vi "Protection Channel.vi"(8 "error in (no error)":errorcluster, 11 "Node Ptr":T2 format="%.0x") -> (0 "error out":errorcluster)   [LabVIEW 2015, in "J1939 Addon System Explorer.lvlib"]
uses:
  J1939 Addon System Explorer.lvlib
  <vilib>/NI Veristand/Custom Device API/Custom Device Item Ref.ctl
  Protection Support/Source/Shared/Types/Protection Type.ctl
  <vilib>/NI VeriStand/Custom Device API/Custom Device API.lvlib
  Protection Support/Source/System Explorer/Protection and Counter Support System Explorer.lvlib
  Protection Support/Source/Shared/Protection and Counter Support Shared.lvlib
panel:
  in  "Protection Type":T1
  in  "SHDocVw.IWebBrowser":refnum<k7>(container)
  in  "Monitored Channels":i32(listbox)
  in  "Header":cluster{"Section Name":string}={"Section Name"="Custom Device Item Settings"}
  in  "Description":string
  in  "Name":string
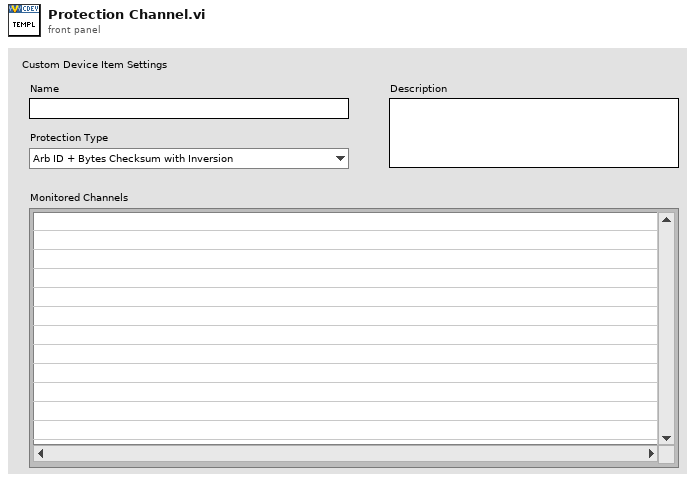
[diagram p1: front panel]
types:
  T1 = typedef "Protection and Counter Support Shared.lvlib/Protection Type.ctl" = enum16{"Arb ID + Bytes Checksum with Inversion", "Arb ID + Bytes CRC with Inversion", "Reversed Raw Signal Checksum with Inversion"}
  T2 = typedef "Custom Device API.lvlib/Custom Device Item Ref.ctl" = u64
  T3 = typedef "Custom Device API.lvlib/Custom Device Item Info.ctl" = cluster{"Name":string, "Is Channel":bool, "GUID":string, "Is Waveform":bool}
  T4 = typedef "Protection and Counter Support System Explorer.lvlib/Protection Signal Settings.ctl" = cluster{"Input Channels":T5[], "Protection Type":T1}
  T5 = typedef "Protection and Counter Support System Explorer.lvlib/Protection Signal Linked Channel.ctl" = cluster{"Node Ref":T2}
  T6 = typedef "Custom Device API.lvlib/Custom Device Commands.ctl" = enum16{"Default", "Item renamed", "Shutdown", "Dynamic button pressed"}
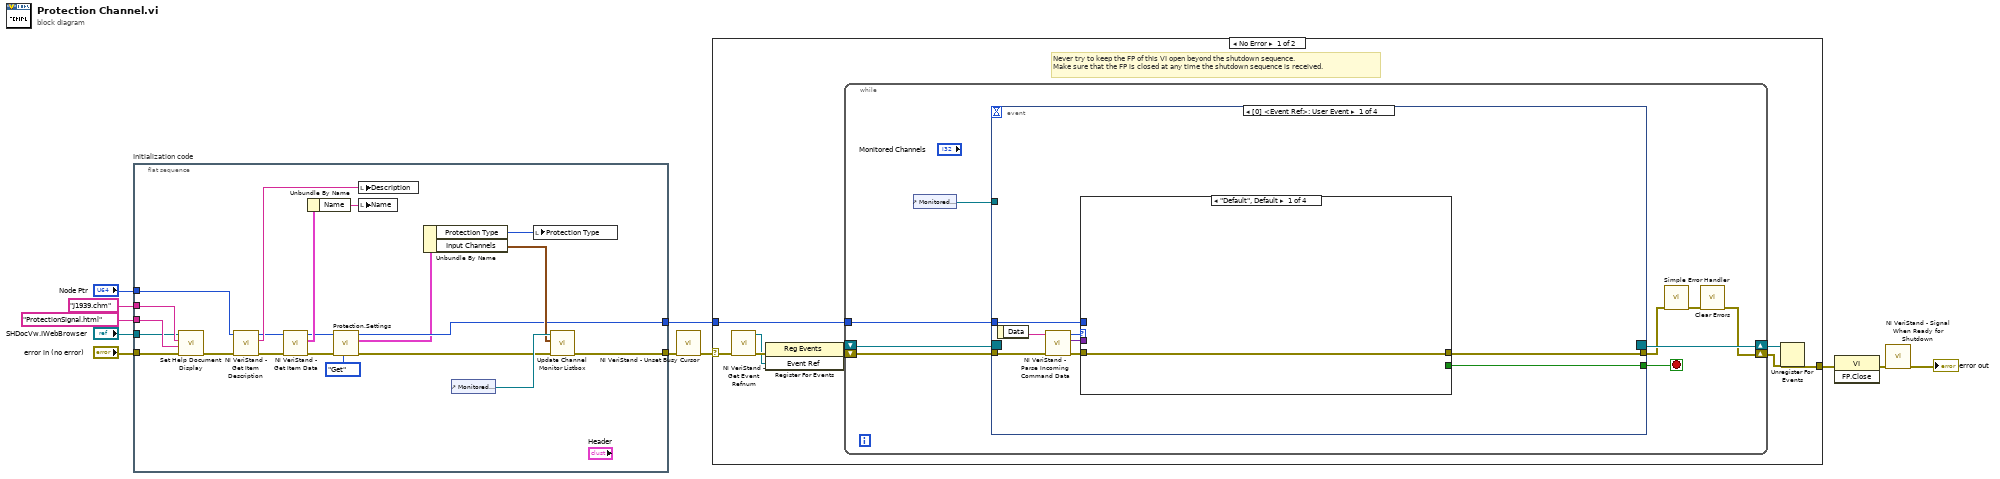
[diagram p0: block diagram]
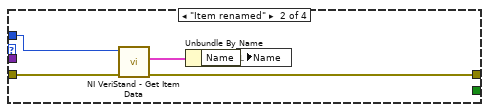
[diagram p2: hidden frame]
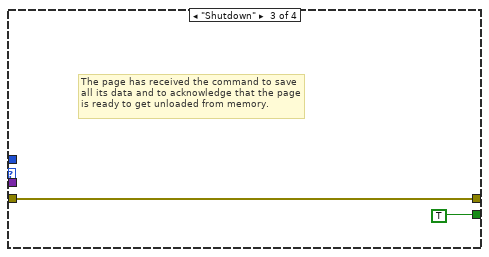
[diagram p3: hidden frame]
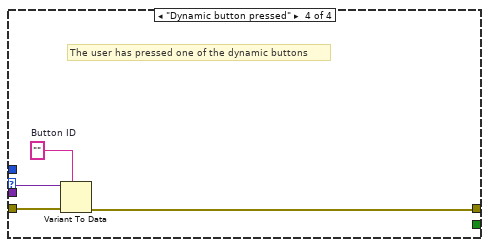
[diagram p4: hidden frame]
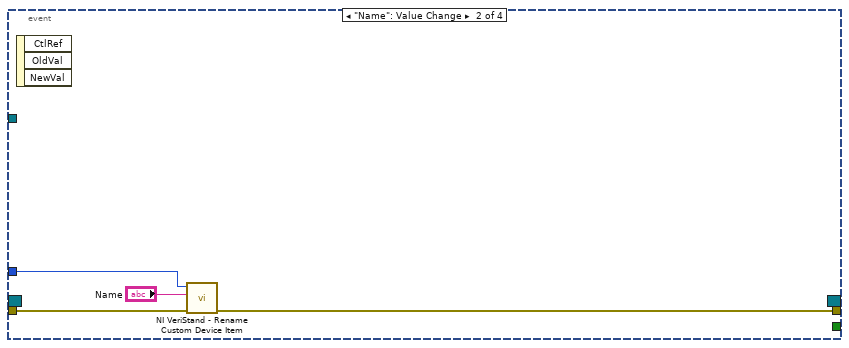
[diagram p5: hidden frame]
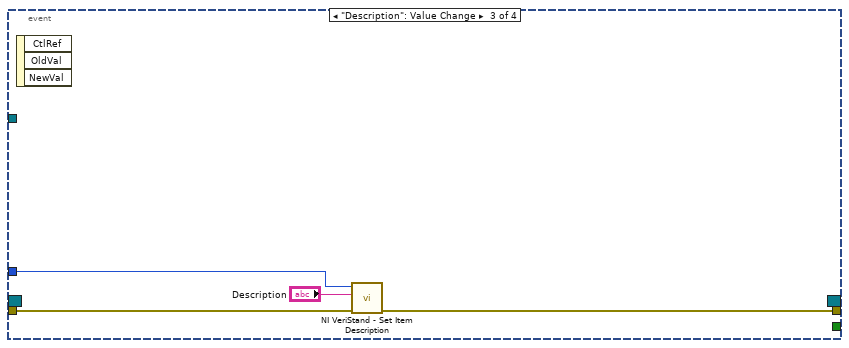
[diagram p6: hidden frame]
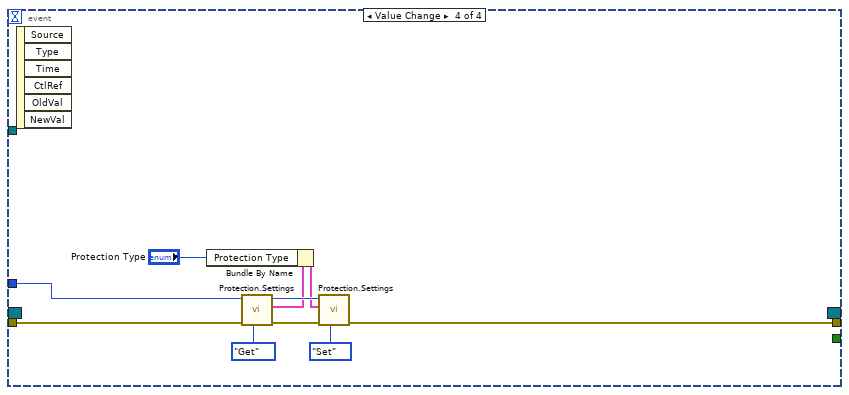
[diagram p7: hidden frame]
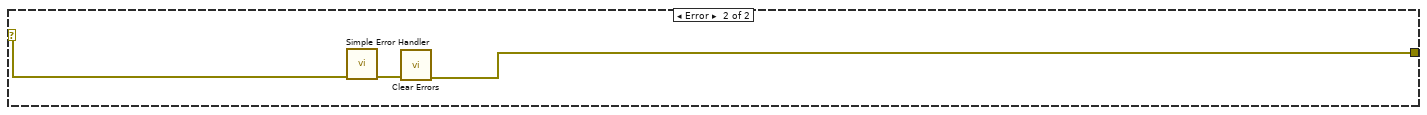
[diagram p8: hidden frame]
diagram:
  n1 = flat-sequence "Initialization code" {
    tunnel: "error in (no error)" -> [w28]
    tunnel: "Node Ptr" -> [w20]
    tunnel: [w13] -> w9
    tunnel: [w15] -> w7
    tunnel: "J1939.chm" ("Main CHM File") -> [w32]
    tunnel: "ProtectionSignal.html" ("HTML File") -> [w31]
    tunnel: "SHDocVw.IWebBrowser" -> [w30]
    frame #0 {
      n2 = call "Set Help Document Display.vi"("error in (no error)"=w28, "HTML File"=w31, "Main CHM File"=w32, "SHDocVw.IWebBrowser2"=w30) -> ("error out"=w21:errorcluster)  [unwired: 7 in]
      n3 = call <vilib>:"NI VeriStand - Get Item Description.vi"("error in (no error)"=w21, "Item Ref in"=w20) -> ("error out"=w24:errorcluster, "Description"=w23:string, "Item Ref out"=w22:T2)  [unwired: 7 out]
      n4 = call <vilib>:"NI VeriStand - Get Item Data.vi"("error in (no error)"=w24, "Item Ref in"=w22) -> ("error out"=w18:errorcluster, "Item Info"=w25:T3, "Item Ref out"=w17:T2)  [unwired: 7 out]
      n5 = Unbundle By Name(w25) -> ("Name"=w26:string)
      n6 = call "Protection.Settings.vi"("Action"=enum8{"Get", "Set"}."Get", "error in"=w18, "Parent Ref"=w17) -> ("error out"=w16:errorcluster, "Selected Channels"=w14:T4, "Parent Ref Out"=w15:T2)  [unwired: 6 in]
      n7 = local write "Description"(w23) -> ()
      n8 = local write "Name"(w26) -> ()
      n9 = Unbundle By Name(w14) -> ("Protection Type"=w19:T1, "Input Channels"=w27:T5[])
      n10 = control-ref of="Monitored Channels"() -> (w29:refnum<vi>)
      n11 = local write "Protection Type"(w19) -> ()
      n12 = call "Update Channel Monitor Listbox.vi"("error in (no error)"=w16, "Input Channels"=w27, "Monitored Channels"=w29) -> ("error out"=w13:errorcluster)  [unwired: 8 in]
    }
  }
  n13 = call <vilib>:"NI VeriStand - Unset Busy Cursor.vi"("error in (no error)"=w9) -> ("error out"=w8:errorcluster)  [unwired: 10 out]
  n14 = case shown="No Error" w8 {
    selector: w8 -> [w33 w91]
    tunnel: [w38 w89] -> w11
    tunnel: w7 -> [w34 _]
    frame No Error {
      # "Never try to keep the FP of this VI open beyond the shutdown sequence.\nMake sure that the FP is closed at any time the shutdown sequence is received."
      n15 = call <vilib>:"NI VeriStand - Get Event Refnum.vi"("error in (no error)"=w33) -> ("error out"=w41:errorcluster, "Event Ref"=w37:refnum<user-event>)  [unwired: 9 out]
      n16 = register-events(error in=w41, w37) -> (reference out=w35:refnum<event-registration>, error out=w36:errorcluster)  [unwired: 1 in]
      n17 = while {
        tunnel: w34 -> [w46]
        shift-right: [w43] -> w39
        shift-left: w36 -> [w49]
        shift-right: [w50] -> w40
        shift-left: w35 -> [w48]
        stop <- w47 stop-if-true
        n18 = control-ref of="Monitored Channels"() -> (w42:refnum<vi>)
        n19 = event shown="[0] <Event Ref>: User Event" {
          selector: w48 -> [_ _ _ _]
          dyn-events: [_ _ _ _] -> w50
          timeout: _ -> [_ _ _ _]
          tunnel: w49 -> [w58 w73 w77 w87]
          tunnel: [w54 _ _ _] -> w47
          tunnel: [w53 w71 w76 w81] -> w45
          tunnel: w46 -> [w52 w72 w75 w88]
          tunnel: w42 -> [_ _ _ _]
          event User Event {
            n20 = event-data() -> ("Data"=w57:string)  [unwired: 1 out]
            n21 = call <vilib>:"NI VeriStand - Parse Incoming Command Data.vi"("error in (no error)"=w58, "Incoming data"=w57) -> ("error out"=w56:errorcluster, "Outgoing data"=w51:variant, "Action"=w55:T6)  [unwired: 7 out]
            n22 = case shown="\"Default\", Default" w55 {
              tunnel: w56 -> [w59 w62 w65 w70]
              tunnel: [_ _ TRUE _] -> w54
              tunnel: [w59 w61 w65 w67] -> w53
              tunnel: w52 -> [_ w60 _ _]
              tunnel: w51 -> [_ _ _ w69]
              frame "Default", Default {
              }
              frame "Item renamed" {
                n23 = call <vilib>:"NI VeriStand - Get Item Data.vi"("error in (no error)"=w62, "Item Ref in"=w60) -> ("error out"=w61:errorcluster, "Item Info"=w63:T3)  [unwired: 8 out]
                n24 = Unbundle By Name(w63) -> ("Name"=w64:string)
                n25 = local write "Name"(w64) -> ()
              }
              frame "Shutdown" {
                # "The page has received the command to save all its data and to acknowledge that the page is ready to get unloaded from memory."
              }
              frame "Dynamic button pressed" {
                w68 = ""  # Button ID
                # "The user has pressed one of the dynamic buttons"
                n26 = Variant To Data(error in=w70, type=w68, Variant=w69) -> (error out=w67:errorcluster)  [unwired: 1 out]
              }
            }
          }
          event "Name": Value Change {
            n27 = event-data() -> ()  [unwired: 4 out]
            n28 = call <vilib>:"NI VeriStand - Rename Custom Device Item.vi"("error in (no error)"=w73, "New Name"="Name", "Item Ref in"=w72) -> ("error out"=w71:errorcluster)  [unwired: 1 in, 7 out]
          }
          event "Description": Value Change {
            n29 = event-data() -> ()  [unwired: 4 out]
            n30 = call <vilib>:"NI VeriStand - Set Item Description.vi"("error in (no error)"=w77, "Description"="Description", "Item Ref in"=w75) -> ("error out"=w76:errorcluster)  [unwired: 8 out]
          }
          event Value Change {
            n31 = event-data() -> ()  [unwired: 7 out]
            n32 = call "Protection.Settings.vi"("Action"=enum8{"Get", "Set"}."Get", "error in"=w87, "Parent Ref"=w88) -> ("error out"=w83:errorcluster, "Selected Channels"=w85:T4, "Parent Ref Out"=w86:T2)  [unwired: 6 in]
            n33 = Bundle By Name(cluster=w85, "Protection Type"="Protection Type") -> (w84:T4)
            n34 = call "Protection.Settings.vi"("Action"=enum8{"Get", "Set"}."Set", "error in"=w83, "Selected Channels"=w84, "Parent Ref"=w86) -> ("error out"=w81:errorcluster)  [unwired: 5 in, 2 out]
          }
        }
        n35 = call <vilib>:"Simple Error Handler.vi"("error in (no error)"=w45) -> ("error out"=w44:errorcluster)  [unwired: 1 in, 7 out]
        n36 = call <vilib>:"Clear Errors.vi"("error in (no error)"=w44) -> ("error out"=w43:errorcluster)  [unwired: 1 in, 5 out]
      }
      n37 = Unregister For Events(event registration refnum=w40, error in=w39) -> (error out=w38:errorcluster)
    }
    frame Error {
      n38 = call <vilib>:"Simple Error Handler.vi"("error in (no error)"=w91) -> ("error out"=w90:errorcluster)  [unwired: 1 in, 7 out]
      n39 = call <vilib>:"Clear Errors.vi"("error in (no error)"=w90) -> ("error out"=w89:errorcluster)  [unwired: 1 in, 5 out]
    }
  }
  n40 = invoke class="VI" method="FP.Close"(error in=w11) -> (error out=w10:errorcluster)  [unwired: 2 in, 2 out]
  n41 = call <vilib>:"NI VeriStand - Signal When Ready for Shutdown.vi"("error in (no error)"=w10) -> ("error out"=→"error out":errorcluster)  [unwired: 10 out]
